vi "WPI_ADI_IMU_Get Angles.vi"(8 "error in":errorcluster, 11 "ADIIMUDevRef":T2 {"Sample Rate" min=0.25 max=100.0 step=0.25}) -> (0 "error out":errorcluster, 2 "IMU Angles":T1, 3 "ADIIMUDevRef":T2 {"Sample Rate" min=0.25 max=100.0 step=0.25})   [LabVIEW 2015, in "FRC ADI MXP IMU.lvlib"]
doc: "Read accumulated angles from the Analog Devices IMU MXP board. Requires the IMU_Loop VI to be running in Periodic Tasks."
uses:
  FRC ADI MXP IMU.lvlib
  WPI_AnalogDevicesIMUDevRef.ctl
  <vilib>/Rock Robotics/SystemInterfaces/spilib/spi_bus.ctl
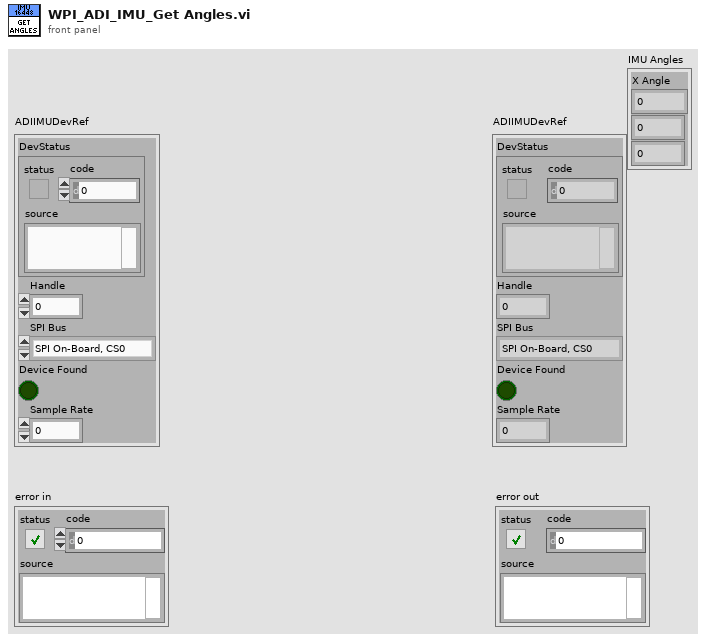
[diagram p1: front panel]
types:
  T1 = cluster{"X Angle":dbl, "Y Angle":dbl, "Z Angle":dbl}
  T2 = typedef "FRC ADI MXP IMU.lvlib/WPI_AnalogDevicesIMUDevRef.ctl" = cluster{"DevStatus":errorcluster, "Handle":i32, "SPI Bus":T3, "Device Found":bool, "Sample Rate":dbl}
  T3 = typedef "spi_bus.ctl" = enum16{"SPI On-Board, CS0", "SPI On-Board, CS1", "SPI On-Board, CS2", "SPI On-Board, CS3", "SPI MXP", "Invalid"}
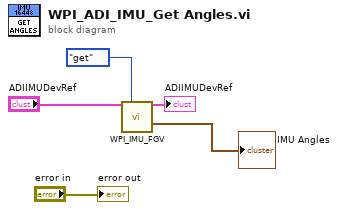
[diagram p0: block diagram]
diagram:
  n1 = call "WPI_IMU_FGV.vi"("SimpleGyroDevRef"="ADIIMUDevRef", "Operation"=enum16{"set", "get"}."get") -> ("SimpleGyroDevRef"=→"ADIIMUDevRef":T2, "IMU Angles Out"=→"IMU Angles":T1)  [unwired: 9 in, 3 out]
  "error out" <- "error in"
